vi "Func-엑셀 데이터를 그래프로 출력.vi"() -> ()   [LabVIEW 2015] (continued)
\n397.98\n397.99\n398.01\n398.03\n398.04\n398.06\n398.08\n398.09\n398.11\n398.13\n398.14\n398.16\n398.18\n398.19\n398.21\n398.23\n398.24\n398.26\n398.28\n398.29\n398.31\n398.33\n398.34\n398.36\n398.38\n398.39\n398.41\n398.43\n398.44\n398.46\n398.48\n398.49\n398.51\n398.53\n398.54\n398.56\n398.58\n398.59\n398.61\n398.63\n398.64\n398.66\n398.68\n398.69\n398.71\n398.73\n398.74\n398.76\n398.78\n398.8\n398.81\n398.83\n398.84\n398.86\n398.88\n398.89\n398.91\n398.93\n398.94\n398.96\n398.98\n398.99\n399.01\n399.03\n399.04\n399.06\n399.08\n399.09\n399.11\n399.13\n399.15\n399.16\n399.18\n399.19\n399.21\n399.23\n399.24\n399.26\n399.28\n399.29\n399.31\n399.33\n399.34\n399.36\n399.38\n399.39\n399.41\n399.43\n399.44\n399.46\n399.48\n399.5\n399.51\n399.53\n399.54\n399.56\n399.58\n399.6\n399.61\n399.63\n399.64\n399.66\n399.68\n399.69\n399.71\n399.73\n399.74\n399.76\n399.78\n399.79\n399.81\n399.83\n399.85\n399.86\n399.88\n399.89\n399.91\n399.93\n399.95\n399.96\n399.98\n399.99\n400.01\n400.03\n400.04\n400.06\n400.08\n400.09\n400.11\n400.13\n400.14\n400.16\n400.18\n400.2\n400.21\n400.23\n400.24\n400.26\n400.28\n400.3\n400.31\n400.33\n400.34\n400.36\n400.38\n400.39\n400.41\n400.43\n400.45\n400.46\n400.48\n400.49\n400.51\n400.53\n400.54\n400.56\n400.58\n400.59\n400.61\n400.63\n400.64\n400.66\n400.68\n400.69\n400.71\n400.73\n400.74\n400.76\n400.78\n400.79\n400.81\n400.83\n400.84\n400.86\n400.88\n400.89\n400.91\n400.93\n400.94\n400.96\n400.98\n400.99\n401.01\n401.03\n401.04\n401.06\n401.08\n401.09\n401.11\n401.13\n401.14\n401.16\n401.18\n401.19\n401.21\n401.23\n401.24\n401.26\n401.28\n401.29\n401.31\n401.33\n401.34\n401.36\n401.38\n401.39\n401.41\n401.43\n401.44\n401.46\n401.48\n401.49\n401.51\n401.53\n401.54\n401.56\n401.58\n401.59\n401.61\n401.63\n401.64\n401.66\n401.68\n401.69\n401.71\n401.73\n401.74\n401.76\n401.78\n401.79\n401.81\n401.83\n401.84\n401.86\n401.88\n401.89\n401.91\n401.93\n401.94\n401.96\n401.98\n401.99\n402.01\n402.03\n402.04\n402.06\n402.08\n402.09\n402.11\n402.13\n402.14\n402.16\n402.18\n402.19\n402.21\n402.23\n402.25\n402.26\n402.28\n402.29\n402.31\n402.33\n402.34\n402.36\n402.38\n402.39\n402.41\n402.43\n402.44\n402.46\n402.48\n402.49\n402.51\n402.53\n402.54\n402.56\n402.58\n402.6\n402.61\n402.63\n402.64\n402.66\n402.68\n402.69\n402.71\n402.73\n402.74\n402.76\n402.78\n402.79\n402.81\n402.83\n402.85\n402.86\n402.88\n402.89\n402.91\n402.93\n402.95\n402.96\n402.98\n402.99\n403.01\n403.03\n403.05\n403.06\n403.08\n403.09\n403.11\n403.13\n403.14\n403.16\n403.18\n403.2\n403.21\n403.23\n403.24\n403.26\n403.28\n403.3\n403.31\n403.33\n403.34\n403.36\n403.38\n403.4\n403.41\n403.43\n403.44\n403.46\n403.48\n403.49\n403.51\n403.53\n403.55\n403.56\n403.58\n403.59\n403.61\n403.63\n403.64\n403.66\n403.68\n403.69\n403.71\n403.73\n403.74\n403.76\n403.78\n403.8\n403.81\n403.83\n403.85\n403.86\n403.88\n403.89\n403.91\n403.93\n403.94\n403.96\n403.98\n403.99\n404.01\n404.03\n404.04\n404.06\n404.08\n404.1\n404.11\n404.13\n404.14\n404.16\n404.18\n404.19\n404.21\n404.23\n404.24\n404.26\n404.28\n404.29\n404.31\n404.33\n404.34\n404.36\n404.38\n404.39\n404.41\n404.43\n404.44\n404.46\n404.48\n404.49\n404.51\n404.53\n404.54\n404.56\n404.58\n404.59\n404.61\n404.63\n404.64\n404.66\n404.68\n404.69\n404.71\n404.73\n404.74\n404.76\n404.78\n404.79\n404.81\n404.83\n404.84\n404.86\n404.88\n404.89\n404.91\n404.93\n404.94\n404.96\n404.98\n405\n405.01\n405.03\n405.04\n405.06\n405.08\n405.09\n405.11\n405.13\n405.14\n405.16\n405.18\n405.19\n405.21\n405.23\n405.24\n405.26\n405.28\n405.29\n405.31\n405.33\n405.35\n405.36\n405.38\n405.39\n405.41\n405.43\n405.44\n405.46\n405.48\n405.49\n405.51\n405.53\n405.54\n405.56\n405.58\n405.59\n405.61\n405.63\n405.64\n405.66\n405.68\n405.7\n405.71\n405.73\n405.74\n405.76\n405.78\n405.8\n405.81\n405.83\n405.84\n405.86\n405.88\n405.89\n405.91\n405.93\n405.95\n405.96\n405.98\n405.99\n406.01\n406.03\n406.05\n406.06\n406.08\n406.09\n406.11\n406.13\n406.14\n406.16\n406.18\n406.19\n406.21\n406.23\n406.24\n406.26\n406.28\n406.3\n406.31\n406.33\n406.34\n406.36\n406.38\n406.4\n406.41\n406.43\n406.44\n406.46\n406.48\n406.49\n406.51\n406.53\n406.54\n406.56\n406.58\n406.59\n406.61\n406.63\n406.65\n406.66\n406.68\n406.69\n406.71\n406.73\n406.74\n406.76\n406.78\n406.79\n406.81\n406.83\n406.84\n406.86\n406.88\n406.89\n406.91\n406.93\n406.94\n406.96\n406.98\n406.99\n407.01\n407.03\n407.04\n407.06\n407.08\n407.09\n407.11\n407.13\n407.14\n407.16\n407.18\n407.19\n407.21\n407.23\n407.24\n407.26\n407.28\n407.29\n407.31\n407.33\n407.34\n407.36\n407.38\n407.39\n407.41\n407.43\n407.44\n407.46\n407.48\n407.49\n407.51\n407.53\n407.54\n407.56\n407.58\n407.59\n407.61\n407.63\n407.64\n407.66\n407.68\n407.69\n407.71\n407.73\n407.74\n407.76\n407.78\n407.79\n407.81\n407.83\n407.84\n407.86\n407.88\n407.89\n407.91\n407.93\n407.94\n407.96\n407.98\n407.99\n408.01\n408.03\n408.04\n408.06\n408.08\n408.1\n408.11\n408.13\n408.14\n408.16\n408.18\n408.19\n408.21\n408.23\n408.24\n408.26\n408.28\n408.29\n408.31\n408.33\n408.34\n408.36\n408.38\n408.39\n408.41\n408.43\n408.45\n408.46\n408.48\n408.49\n408.51\n408.53\n408.54\n408.56\n408.58\n408.59\n408.61\n408.63\n408.64\n408.66\n408.68\n408.69\n408.71\n408.73\n408.74\n408.76\n408.78\n408.8\n408.81\n408.83\n408.84\n408.86\n408.88\n408.89\n408.91\n408.93\n408.94\n408.96\n408.98\n408.99\n409.01\n409.03\n409.05\n409.06\n409.08\n409.09\n409.11\n409.13\n409.15\n409.16\n409.18\n409.19\n409.21\n409.23\n409.24\n409.26\n409.28\n409.29\n409.31\n409.33\n409.34\n409.36\n409.38\n409.4\n409.41\n409.43\n409.44\n409.46\n409.48\n409.49\n409.51\n409.53\n409.54\n409.56\n409.58\n409.59\n409.61\n409.63\n409.64\n409.66\n409.68\n409.69\n409.71\n409.73\n409.75\n409.76\n409.78\n409.79\n409.81\n409.83\n409.84\n409.86\n409.88\n409.89\n409.91\n409.93\n409.94\n409.96\n409.98\n409.99\n410.01\n410.03\n410.04\n410.06\n410.08\n410.09\n410.11\n410.13\n410.14\n410.16\n410.18\n410.19\n410.21\n410.23\n410.24\n410.26\n410.28\n410.29\n410.31\n410.33\n410.34\n410.36\n410.38\n410.39\n410.41\n410.43\n410.45\n410.46\n410.48\n410.49\n410.51\n410.53\n410.54\n410.56\n410.58\n410.59\n410.61\n410.63\n410.64\n410.66\n410.68\n410.69\n410.71\n410.73\n410.74\n410.76\n410.78\n410.79\n410.81\n410.83\n410.84\n410.86\n410.88\n410.89\n410.91\n410.93\n410.94\n410.96\n410.98\n410.99\n411.01\n411.03\n411.04\n411.06\n411.08\n411.09\n411.11\n411.13\n411.14\n411.16\n411.18\n411.19\n411.21\n411.23\n411.24\n411.26\n411.28\n411.29\n411.31\n411.33\n411.34\n411.36\n411.38\n411.39\n411.41\n411.43\n411.44\n411.46\n411.48\n411.49\n411.51\n411.53\n411.55\n411.56\n411.58\n411.59\n411.61\n411.63\n411.64\n411.66\n411.68\n411.69\n411.71\n411.73\n411.74\n411.76\n411.78\n411.8\n411.81\n411.83\n411.84\n411.86\n411.88\n411.9\n411.91\n411.93\n411.94\n411.96\n411.98\n411.99\n412.01\n412.03\n412.04\n412.06\n412.08\n412.09\n412.11\n412.13\n412.15\n412.16\n412.18\n412.19\n412.21\n412.23\n412.25\n412.26\n412.28\n412.29\n412.31\n412.33\n412.34\n412.36\n412.38\n412.39\n412.41\n412.43\n412.44\n412.46\n412.48\n412.5\n412.51\n412.53\n412.54\n412.56\n412.58\n412.6\n412.61\n412.63\n412.64\n412.66\n412.68\n412.69\n412.71\n412.73\n412.75\n412.76\n412.78\n412.79\n412.81\n412.83\n412.84\n412.86\n412.88\n412.89\n412.91\n412.93\n412.94\n412.96\n412.98\n412.99\n413.01\n413.03\n413.04\n413.06\n413.08\n413.09\n413.11\n413.13\n413.14\n413.16\n413.18\n413.2\n413.21\n413.23\n413.24\n413.26\n413.28\n413.29\n413.31\n413.33\n413.34\n413.36\n413.38\n413.39\n413.41\n413.43\n413.44\n413.46\n413.48\n413.49\n413.51\n413.53\n413.54\n413.56\n413.58\n413.59\n413.61\n413.63\n413.64\n413.66\n413.68\n413.69\n413.71\n413.73\n413.74\n413.76\n413.78\n413.79\n413.81\n413.83\n413.84\n413.86\n413.88\n413.89\n413.91\n413.93\n413.94\n413.96\n413.98\n413.99\n414.01\n414.03\n414.04\n414.06\n414.08\n414.09\n414.11\n414.13\n414.14\n414.16\n414.18\n414.19\n414.21\n414.23\n414.24\n414.26\n414.28\n414.29\n414.31\n414.33\n414.34\n414.36\n414.38\n414.39\n414.41\n414.43\n414.44\n414.46\n414.48\n414.49\n414.51\n414.53\n414.54\n414.56\n414.58\n414.59\n414.61\n414.63\n414.64\n414.66\n414.68\n414.69\n414.71\n414.73\n414.74\n414.76\n414.78\n414.79\n414.81\n414.83\n414.84\n414.86\n414.88\n414.9\n414.91\n414.93\n414.94\n414.96\n414.98\n415\n415.01\n415.03\n415.04\n415.06\n415.08\n415.09\n415.11\n415.13\n415.14\n415.16\n415.18\n415.19\n415.21\n415.23\n415.25\n415.26\n415.28\n415.29\n415.31\n415.33\n415.35\n415.36\n415.38\n415.39\n415.41\n415.43\n415.44\n415.46\n415.48\n415.5\n415.51\n415.53\n415.54\n415.56\n415.58\n415.6\n415.61\n415.63\n415.64\n415.66\n415.68\n415.7\n415.71\n415.73\n415.74\n415.76\n415.78\n415.79\n415.81\n415.83\n415.84\n415.86\n415.88\n415.89\n415.91\n415.93\n415.94\n415.96\n415.98\n415.99\n416.01\n416.03\n416.04\n416.06\n416.08\n416.09\n416.11\n416.13\n416.14\n416.16\n416.18\n416.19\n416.21\n416.23\n416.24\n416.26\n416.28\n416.29\n416.31\n416.33\n416.34\n416.36\n416.38\n416.39\n416.41\n416.43\n416.45\n416.46\n416.48\n416.49\n416.51\n416.53\n416.54\n416.56\n416.58\n416.59\n416.61\n416.63\n416.64\n416.66\n416.68\n416.69\n416.71\n416.73\n416.74\n416.76\n416.78\n416.79\n416.81\n416.83\n416.84\n416.86\n416.88\n416.89\n416.91\n416.93\n416.94\n416.96\n416.98\n416.99\n417.01\n417.03\n417.04\n417.06\n417.08\n417.09\n417.11\n417.13\n417.14\n417.16\n417.18\n417.19\n417.21\n417.23\n417.24\n417.26\n417.28\n417.29\n417.31\n417.33\n417.34\n417.36\n417.38\n417.39\n417.41\n417.43\n417.44\n417.46\n417.48\n417.49\n417.51\n417.53\n417.54\n417.56\n417.58\n417.59\n417.61\n417.63\n417.65\n417.66\n417.68\n417.69\n417.71\n417.73\n417.75\n417.76\n417.78\n417.79\n417.81\n417.83\n417.84\n417.86\n417.88\n417.89\n417.91\n417.93\n417.94\n417.96\n417.98\n418\n418.01\n418.03\n418.04\n418.06\n418.08\n418.1\n418.11\n418.13\n418.14\n418.16\n418.18\n418.19\n418.21\n418.23\n418.25\n418.26\n418.28\n418.29\n418.31\n418.33\n418.35\n418.36\n418.38\n418.39\n418.41\n418.43\n418.45\n418.46\n418.48\n418.49\n418.51\n418.53\n418.54\n418.56\n418.58\n418.59\n418.61\n418.63\n418.64\n418.66\n418.68\n418.7\n418.71\n418.73\n418.74\n418.76\n418.78\n418.8\n418.81\n418.83\n418.84\n418.86\n418.88\n418.89\n418.91\n418.93\n418.95\n418.96\n418.98\n418.99\n419.01\n419.03\n419.04\n419.06\n419.08\n419.09\n419.11\n419.13\n419.15\n419.16\n419.18\n419.19\n419.21\n419.23\n419.24\n419.26\n419.28\n419.29\n419.31\n419.33\n419.34\n419.36\n419.38\n419.39\n419.41\n419.43\n419.44\n419.46\n419.48\n419.49\n419.51\n419.53\n419.54\n419.56\n419.58\n419.59\n419.61\n419.63\n419.64\n419.66\n419.68\n419.69\n419.71\n419.73\n419.74\n419.76\n419.78\n419.79\n419.81\n419.83\n419.84\n419.86\n419.88\n419.89\n419.91\n419.93\n419.94\n419.96\n419.98\n419.99\n420.01\n420.03\n420.04\n420.06\n420.08\n420.09\n420.11\n420.13\n420.14\n420.16\n420.18\n420.19\n420.21\n420.23\n420.24\n420.26\n420.28\n420.29\n420.31\n420.33\n420.34\n420.36\n420.38\n420.39\n420.41\n420.43\n420.44\n420.46\n420.48\n420.49\n420.51\n420.53\n420.54\n420.56\n420.58\n420.59\n420.61\n420.63\n420.64\n420.66\n420.68\n420.69\n420.71\n420.73\n420.75\n420.76\n420.78\n420.79\n420.81\n420.83\n420.85\n420.86\n420.88\n420.89\n420.91\n420.93\n420.94\n420.96\n420.98\n420.99\n421.01\n421.03\n421.04\n421.06\n421.08\n421.1\n421.11\n421.13\n421.14\n421.16\n421.18\n421.19\n421.21\n421.23\n421.24\n421.26\n421.28\n421.29\n421.31\n421.33\n421.34\n421.36\n421.38\n421.39\n421.41\n421.43\n421.44\n421.46\n421.48\n421.49\n421.51\n421.53\n421.54\n421.56\n421.58\n421.59\n421.61\n421.63\n421.64\n421.66\n421.68\n421.69\n421.71\n421.73\n421.74\n421.76\n421.78\n421.8\n421.81\n421.83\n421.84\n421.86\n421.88\n421.9\n421.91\n421.93\n421.94\n421.96\n421.98\n421.99\n422.01\n422.03\n422.04\n422.06\n422.08\n422.09\n422.11\n422.13\n422.14\n422.16\n422.18\n422.19\n422.21\n422.23\n422.24\n422.26\n422.28\n422.29\n422.31\n422.33\n422.34\n422.36\n422.38\n422.39\n422.41\n422.43\n422.44\n422.46\n422.48\n422.49\n422.51\n422.53\n422.54\n422.56\n422.58\n422.59\n422.61\n422.63\n422.64\n422.66\n422.68\n422.69\n422.71\n422.73\n422.74\n422.76\n422.78\n422.79\n422.81\n422.83\n422.84\n422.86\n422.88\n422.89\n422.91\n422.93\n422.94\n422.96\n422.98\n422.99\n423.01\n423.03\n423.04\n423.06\n423.08\n423.09\n423.11\n423.13\n423.14\n423.16\n423.18\n423.19\n423.21\n423.23\n423.24\n423.26\n423.28\n423.29\n423.31\n423.33\n423.34\n423.36\n423.38\n423.39\n423.41\n423.43\n423.44\n423.46\n423.48\n423.5\n423.51\n423.53\n423.54\n423.56\n423.58\n423.59\n423.61\n423.63\n423.64\n423.66\n423.68\n423.69\n423.71\n423.73\n423.74\n423.76\n423.78\n423.79\n423.81\n423.83\n423.85\n423.86\n423.88\n423.89\n423.91\n423.93\n423.94\n423.96\n423.98\n423.99\n424.01\n424.03\n424.04\n424.06\n424.08\n424.09\n424.11\n424.13\n424.14\n424.16\n424.18\n424.2\n424.21\n424.23\n424.24\n424.26\n424.28\n424.3\n424.31\n424.33\n424.34\n424.36\n424.38\n424.39\n424.41\n424.43\n424.45\n424.46\n424.48\n424.49\n424.51\n424.53\n424.55\n424.56\n424.58\n424.59\n424.61\n424.63\n424.64\n424.66\n424.68\n424.69\n424.71\n424.73\n424.74\n424.76\n424.78\n424.8\n424.81\n424.83\n424.84\n424.86\n424.88\n424.89\n424.91\n424.93\n424.94\n424.96\n424.98\n425\n425.01\n425.03\n425.04\n425.06\n425.08\n425.09\n425.11\n425.13\n425.14\n425.16\n425.18\n425.19\n425.21\n425.23\n425.24\n425.26\n425.28\n425.29\n425.31\n425.33\n425.34\n425.36\n425.38\n425.39\n425.41\n425.43\n425.44\n425.46\n425.48\n425.49\n425.51\n425.53\n425.54\n425.56\n425.58\n425.6\n425.61\n425.63\n425.64\n425.66\n425.68\n425.69\n425.71\n425.73\n425.74\n425.76\n425.78\n425.79\n425.81\n425.83\n425.84\n425.86\n425.88\n425.89\n425.91\n425.93\n425.94\n425.96\n425.98\n425.99\n426.01\n426.03\n426.04\n426.06\n426.08\n426.09\n426.11\n426.13\n426.14\n426.16\n426.18\n426.19\n426.21\n426.23\n426.24\n426.26\n426.28\n426.29\n426.31\n426.33\n426.34\n426.36\n426.38\n426.39\n426.41\n426.43\n426.44\n426.46\n426.48\n426.49\n426.51\n426.53\n426.54\n426.56\n426.58\n426.59\n426.61\n426.63\n426.64\n426.66\n426.68\n426.69\n426.71\n426.73\n426.74\n426.76\n426.78\n426.79\n426.81\n426.83\n426.84\n426.86\n426.88\n426.89\n426.91\n426.93\n426.95\n426.96\n426.98\n426.99\n427.01\n427.03\n427.04\n427.06\n427.08\n427.09\n427.11\n427.13\n427.14\n427.16\n427.18\n427.19\n427.21\n427.23\n427.24\n427.26\n427.28\n427.3\n427.31\n427.33\n427.34\n427.36\n427.38\n427.39\n427.41\n427.43\n427.44\n427.46\n427.48\n427.49\n427.51\n427.53\n427.54\n427.56\n427.58\n427.59\n427.61\n427.63\n427.65\n427.66\n427.68\n427.69\n427.71\n427.73\n427.74\n427.76\n427.78\n427.79\n427.81\n427.83\n427.84\n427.86\n427.88\n427.9\n427.91\n427.93\n427.94\n427.96\n427.98\n427.99\n428.01\n428.03\n428.04\n428.06\n428.08\n428.1\n428.11\n428.13\n428.14\n428.16\n428.18\n428.19\n428.21\n428.23\n428.25\n428.26\n428.28\n428.29\n428.31\n428.33\n428.34\n428.36\n428.38\n428.39\n428.41\n428.43\n428.44\n428.46\n428.48\n428.49\n428.51\n428.53\n428.54\n428.56\n428.58\n428.59\n428.61\n428.63\n428.64\n428.66\n428.68\n428.69\n428.71\n428.73\n428.74\n428.76\n428.78\n428.79\n428.81\n428.83\n428.84\n428.86\n428.88\n428.89\n428.91\n428.93\n428.94\n428.96\n428.98\n428.99\n429.01\n429.03\n429.04\n429.06\n429.08\n429.09\n429.11\n429.13\n429.14\n429.16\n429.18\n429.19\n429.21\n429.23\n429.24\n429.26\n429.28\n429.29\n429.31\n429.33\n429.34\n429.36\n429.38\n429.39\n429.41\n429.43\n429.44\n429.46\n429.48\n429.49\n429.51\n429.53\n429.54\n429.56\n429.58\n429.59\n429.61\n429.63\n429.64\n429.66\n429.68\n429.69\n429.71\n429.73\n429.74\n429.76\n429.78\n429.79\n429.81\n429.83\n429.84\n429.86\n429.88\n429.89\n429.91\n429.93\n429.94\n429.96\n429.98\n429.99\n430.01\n430.03\n430.05\n430.06\n430.08\n430.09\n430.11\n430.13\n430.14\n430.16\n430.18\n430.19\n430.21\n430.23\n430.24\n430.26\n430.28\n430.3\n430.31\n430.33\n430.34\n430.36\n430.38\n430.4\n430.41\n430.43\n430.44\n430.46\n430.48\n430.49\n430.51\n430.53\n430.54\n430.56\n430.58\n430.59\n430.61\n430.63\n430.65\n430.66\n430.68\n430.69\n430.71\n430.73\n430.75\n430.76\n430.78\n430.79\n430.81\n430.83\n430.85\n430.86\n430.88\n430.9\n430.91\n430.93\n430.94\n430.96\n430.98\n430.99\n431.01\n431.03\n431.04\n431.06\n431.08\n431.1\n431.11\n431.13\n431.14\n431.16\n431.18\n431.19\n431.21\n431.23\n431.25\n431.26\n431.28\n431.29\n431.31\n431.33\n431.34\n431.36\n431.38\n431.39\n431.41\n431.43\n431.44\n431.46\n431.48\n431.49\n431.51\n431.53\n431.54\n431.56\n431.58\n431.59\n431.61\n431.63\n431.64\n431.66\n431.68\n431.69\n431.71\n431.73\n431.74\n431.76\n431.78\n431.79\n431.81\n431.83\n431.84\n431.86\n431.88\n431.89\n431.91\n431.93\n431.94\n431.96\n431.98\n431.99\n432.01\n432.03\n432.04\n432.06\n432.08\n432.09\n432.11\n432.13\n432.14\n432.16\n432.18\n432.19\n432.21\n432.23\n432.24\n432.26\n432.28\n432.29\n432.31\n432.33\n432.34\n432.36\n432.38\n432.39\n432.41\n432.43\n432.44\n432.46\n432.48\n432.49\n432.51\n432.53\n432.54\n432.56\n432.58\n432.59\n432.61\n432.63\n432.64\n432.66\n432.68\n432.69\n432.71\n432.73\n432.74\n432.76\n432.78\n432.79\n432.81\n432.83\n432.84\n432.86\n432.88\n432.89\n432.91\n432.93\n432.94\n432.96\n432.98\n432.99\n433.01\n433.03\n433.05\n433.06\n433.08\n433.09\n433.11\n433.13\n433.14\n433.16\n433.18\n433.19\n433.21\n433.23\n433.24\n433.26\n433.28\n433.29\n433.31\n433.33\n433.34\n433.36\n433.38\n433.4\n433.41\n433.43\n433.44\n433.46\n433.48\n433.5\n433.51\n433.53\n433.54\n433.56\n433.58\n433.59\n450.14\n450.31\n450.47\n450.64\n450.81\n450.97\n451.14\n451.31\n451.47\n451.64\n451.81\n451.97\n452.14\n452.31\n452.47\n452.64\n452.81\n452.97\n453.14\n453.31\n453.47\n453.64\n453.81\n453.97\n454.14\n454.31\n454.47\n454.64\n454.81\n454.97\n455.14\n455.31\n455.47\n455.64\n455.81\n455.97\n456.14\n456.31\n456.48\n456.65\n456.81\n456.98\n457.15\n457.31\n457.48\n457.65\n457.81\n457.98\n458.15\n458.31\n458.48\n458.65\n458.81\n458.98\n459.15\n459.31\n459.48\n459.65\n459.81\n459.98\n460.15\n460.31\n460.48\n460.65\n460.81\n460.98\n461.15\n461.31\n461.48\n461.65\n461.81\n461.98\n462.15\n462.31\n462.48\n462.65\n462.81\n462.98\n463.15\n463.31\n463.48\n463.65\n463.81\n463.98\n464.15\n464.31\n464.48\n464.65\n464.81\n464.98\n465.15\n465.31\n465.48\n465.65\n465.81\n465.98\n466.15\n466.31\n466.48\n466.65\n466.81\n466.98\n467.15\n467.31\n467.48\n467.65\n467.81\n467.98\n468.15\n468.31\n468.48\n468.65\n468.81\n468.98\n469.15\n469.31\n469.48\n469.65\n469.81\n469.98\n470.15\n470.31\n470.48\n470.65\n470.81\n470.98\n471.15\n471.31\n471.48\n471.65\n471.81\n471.99\n472.16\n472.32\n472.49\n472.66\n472.82\n472.99\n473.16\n473.32\n473.49\n473.66\n473.82\n473.99\n474.16\n474.32\n474.49\n474.66\n474.82\n474.99\n475.16\n475.32\n475.49\n475.66\n475.82\n475.99\n476.16\n476.32\n476.49\n476.66\n476.82\n476.99\n477.16\n477.32\n477.49\n477.66\n477.82\n477.99\n478.16\n478.32\n478.49\n478.66\n478.82\n478.99\n479.16\n479.32\n479.49\n479.66\n479.82\n479.99\n480.16\n480.32\n480.49\n480.66\n480.82\n480.99\n481.16\n481.32\n481.49\n481.66\n481.82\n481.99\n482.16\n482.32\n482.49\n482.66\n482.82\n482.99\n483.16\n483.32\n483.49\n483.66\n483.82\n483.99\n484.16\n484.32\n484.49\n484.66\n484.82\n484.99\n485.16\n485.32\n485.49\n485.66\n485.82\n485.99\n486.16\n486.32\n486.49\n486.66\n486.82\n486.99\n487.16\n487.32\n487.49\n487.66\n487.82\n487.99\n488.16\n488.32\n488.49\n488.66\n488.83\n489\n489.16\n489.33\n489.5\n489.66\n489.82\n489.83\n489.84\n489.86\n489.88\n489.89\n489.91\n489.93\n489.94\n489.96\n489.98\n489.99\n490.01\n490.03\n490.04\n490.06\n490.08\n490.09\n490.11\n490.13\n490.14\n490.16\n490.18\n490.19\n490.21\n490.23\n490.24\n490.26\n490.28\n490.29\n490.31\n490.33\n490.34\n490.36\n490.38\n490.39\n490.41\n490.43\n490.44\n490.46\n490.48\n490.49\n490.51\n490.53\n490.54\n490.56\n490.58\n490.6\n490.61\n490.63\n490.64\n490.66\n490.68\n490.69\n490.71\n490.73\n490.74\n490.76\n490.78\n490.79\n490.81\n490.83\n490.85\n490.86\n490.88\n490.89\n490.91\n490.93\n490.94\n490.96\n490.98\n490.99\n491.01\n491.03\n491.04\n491.06\n491.08\n491.09\n491.11\n491.13\n491.14\n491.16\n491.18\n491.2\n491.21\n491.23\n491.24\n491.26\n491.28\n491.3\n491.31\n491.33\n491.34\n491.36\n491.38\n491.39\n491.41\n491.43\n491.44\n491.46\n491.48\n491.49\n491.51\n491.53\n491.55\n491.56\n491.58\n491.59\n491.61\n491.63\n491.65\n491.66\n491.68\n491.69\n491.71\n491.73\n491.74\n491.76\n491.78\n491.79\n491.81\n491.83\n491.84\n491.86\n491.88\n491.89\n491.91\n491.93\n491.94\n491.96\n491.98\n492\n492.01\n
